vi "Get Bitfile Path.vi"(7 "Config Bitfile Path Ref":refnum<vi>, 8 "error in (no error)":errorcluster, 10 "SI Count":i32, 11 "Module Name":string) -> (0 "error out":errorcluster, 3 "Bitfile Path":path)   [LabVIEW 2025, in "I2C Bus Monitor UI.lvlib"]
uses:
  I2C Bus Monitor UI.lvlib
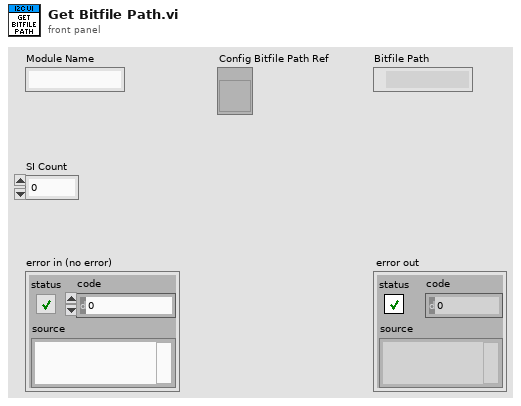
[diagram p1: front panel]
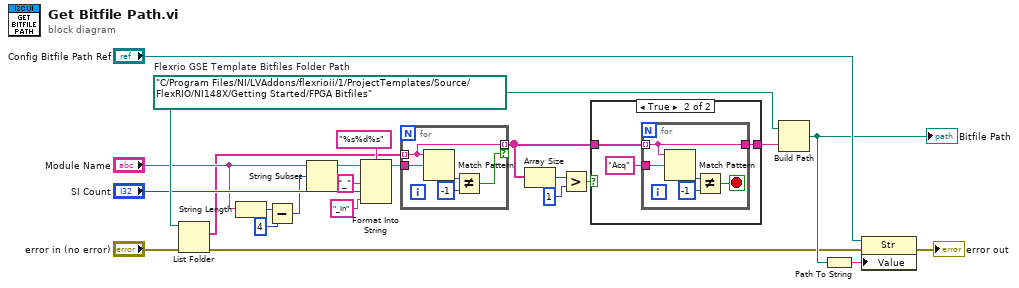
[diagram p0: block diagram]
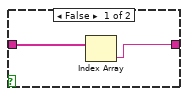
[diagram p2: hidden frame]
diagram:
  w21 = path "C:/Program Files/NI/LVAddons/flexrioii/1/ProjectTemplates/Source/FlexRIO/NI148X/Getting Started/FPGA Bitfiles"  # Flexrio GSE Template Bitfiles Folder Path
  n1 = List Folder(path=w21, error in="error in (no error)") -> (filenames=w6:string[], error out=w2:errorcluster)  [unwired: 2 in, 2 out]
  n2 = String Length(string="Module Name") -> (length=w8:i32)
  n3 = Subtract(x=w8, y=4) -> (x-y=w9:i32)
  n4 = String Subset(string="Module Name", offset (0)=w9) -> (substring=w12:string)  [unwired: 1 in]
  n5 = Format Into String(format string="%s%d%s", initial string=w12, "_" ("substring"), "SI Count", "_In" ("substring")) -> (resulting string=w13:string)  [unwired: 1 in, 1 out]
  n6 = for {
    tunnel: w6 -> [w25] mode=indexing
    tunnel: w13 -> [w28]
    tunnel: [w25] -> w20 mode=indexing if=w24
    n7 = Match Pattern(string=w25, regular expression=w28) -> (offset past match=w26:i32)  [unwired: 1 in, 3 out]
    n8 = Not Equal?(x=w26, y=-1) -> (x != y?=w24:bool)
  }
  n9 = Array Size(array=w20) -> (size(s)=w17:i32)
  n10 = Greater?(x=w17, y=1) -> (0:w19:bool)
  n11 = case shown="True" w19 {
    tunnel: w20 -> [w30 w33]
    tunnel: [w29 w31] -> w22
    frame False {
      n12 = Index Array(array=w30) -> (element=w29:string)  [unwired: 1 in]
    }
    frame True {
      n13 = for {
        tunnel: w33 -> [w35] mode=indexing
        tunnel: "Acq" -> [w38]
        tunnel: [w35] -> w31
        stop <- w34 stop-if-true
        n14 = Match Pattern(string=w35, regular expression=w38) -> (offset past match=w36:i32)  [unwired: 1 in, 3 out]
        n15 = Not Equal?(x=w36, y=-1) -> (x != y?=w34:bool)
      }
    }
  }
  n16 = Build Path(base path=w21, name or relative path=w22) -> (appended path=w4:path)
  "Bitfile Path" <- w4
  n17 = Path To String(path=w4) -> (string=w3:string)
  n18 = property class="Str"(reference="Config Bitfile Path Ref", error in=w2, "Value"=w3) -> (error out=→"error out":errorcluster)  [unwired: 1 out]
